vi "ZoneBlue rotatePlace.vi"   [LabVIEW 2019]
uses:
  Global Var.vi
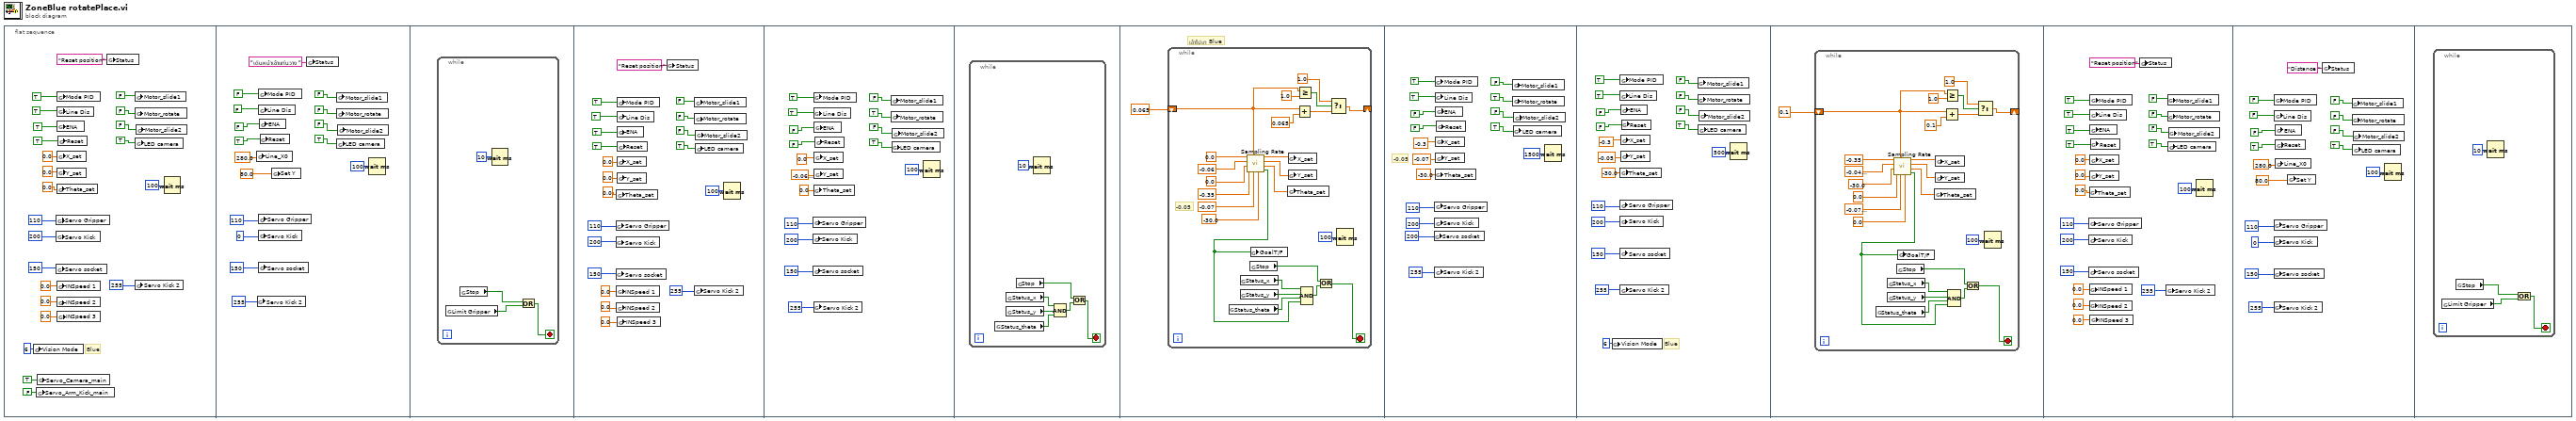
[diagram p0: block diagram]
diagram:
  n1 = flat-sequence {
    frame #0 {
      # "Blue"
      n2 = global write "Global Var.vi" "Vision Mode"(i16 6 ("Vision Mode")) -> ()
      n3 = global write "Global Var.vi" "Servo_Arm_Kick_main"(FALSE ("Mode PID")) -> ()
      n4 = global write "Global Var.vi" "Servo_Camera_main"(TRUE ("Mode PID")) -> ()
      n5 = global write "Global Var.vi" "Servo Gripper"(u8 110 ("Servo Camera")) -> ()
      n6 = global write "Global Var.vi" "Servo Kick"(u8 200 ("Servo Camera")) -> ()
      n7 = global write "Global Var.vi" "Servo socket"(u8 150 ("Servo Camera")) -> ()
      n8 = global write "Global Var.vi" "Theta_set"(0.0 ("Theta_set")) -> ()
      n9 = global write "Global Var.vi" "INSpeed 1"(0.0 ("X_set")) -> ()
      n10 = global write "Global Var.vi" "INSpeed 2"(0.0 ("Y_set")) -> ()
      n11 = global write "Global Var.vi" "Mode PID"(TRUE ("Mode PID")) -> ()
      n12 = global write "Global Var.vi" "Line Dis"(TRUE ("Mode PID")) -> ()
      n13 = global write "Global Var.vi" "ENA"(TRUE ("ENA")) -> ()
      n14 = global write "Global Var.vi" "X_set"(0.0 ("X_set")) -> ()
      n15 = global write "Global Var.vi" "Y_set"(0.0 ("Y_set")) -> ()
      n16 = global write "Global Var.vi" "INSpeed 3"(0.0 ("Theta_set")) -> ()
      n17 = global write "Global Var.vi" "Reset"(TRUE ("ENA")) -> ()
      n18 = global write "Global Var.vi" "Status"("Reset position" ("Status")) -> ()
      n19 = global write "Global Var.vi" "Motor_slide1"(FALSE ("Mode PID")) -> ()
      n20 = global write "Global Var.vi" "Motor_rotate"(FALSE ("ENA")) -> ()
      n21 = global write "Global Var.vi" "Servo Kick 2"(u8 255 ("Servo Camera")) -> ()
      n22 = global write "Global Var.vi" "LED camera"(TRUE ("LED camera")) -> ()
      n23 = global write "Global Var.vi" "Motor_slide2"(FALSE ("ENA")) -> ()
      n24 = Wait (ms)(milliseconds to wait=u32 100) -> ()  [unwired: 1 out]
    }
    frame #1 {
      n25 = global write "Global Var.vi" "Line_X0"(280.0 ("Y_set")) -> ()
      n26 = global write "Global Var.vi" "Servo Kick 2"(u8 255 ("Servo Camera")) -> ()
      n27 = global write "Global Var.vi" "Servo Gripper"(u8 110 ("Servo Camera")) -> ()
      n28 = global write "Global Var.vi" "Servo Kick"(u8 0 ("Servo Camera")) -> ()
      n29 = global write "Global Var.vi" "Servo socket"(u8 150 ("Servo Camera")) -> ()
      n30 = global write "Global Var.vi" "Mode PID"(FALSE ("Mode PID")) -> ()
      n31 = global write "Global Var.vi" "Line Dis"(FALSE ("Mode PID")) -> ()
      n32 = global write "Global Var.vi" "ENA"(FALSE ("ENA")) -> ()
      n33 = global write "Global Var.vi" "Reset"(TRUE ("ENA")) -> ()
      n34 = global write "Global Var.vi" "Set Y"(80.0 ("Y_set")) -> ()
      n35 = global write "Global Var.vi" "Status"("เดินหน้าเข้าแท่นวาง " ("Status")) -> ()
      n36 = global write "Global Var.vi" "Motor_slide1"(FALSE ("Mode PID")) -> ()
      n37 = global write "Global Var.vi" "Motor_rotate"(FALSE ("ENA")) -> ()
      n38 = global write "Global Var.vi" "LED camera"(TRUE ("LED camera")) -> ()
      n39 = global write "Global Var.vi" "Motor_slide2"(FALSE ("ENA")) -> ()
      n40 = Wait (ms)(milliseconds to wait=u32 100) -> ()  [unwired: 1 out]
    }
    frame #2 {
      n41 = while {
        stop <- w42 stop-if-true
        n42 = global read "Global Var.vi" "Limit Gripper"() -> (w40:bool)
        n43 = global read "Global Var.vi" "Stop"() -> (w41:bool)
        n44 = Wait (ms)(milliseconds to wait=u32 10) -> ()  [unwired: 1 out]
        n45 = Or(x=w41, y=w40) -> (x .or. y?=w42:bool)
      }
    }
    frame #3 {
      n46 = global write "Global Var.vi" "Servo Gripper"(u8 110 ("Servo Camera")) -> ()
      n47 = global write "Global Var.vi" "Servo Kick"(u8 200 ("Servo Camera")) -> ()
      n48 = global write "Global Var.vi" "Servo socket"(u8 150 ("Servo Camera")) -> ()
      n49 = global write "Global Var.vi" "Theta_set"(0.0 ("Theta_set")) -> ()
      n50 = global write "Global Var.vi" "INSpeed 1"(0.0 ("X_set")) -> ()
      n51 = global write "Global Var.vi" "INSpeed 2"(0.0 ("Y_set")) -> ()
      n52 = global write "Global Var.vi" "Mode PID"(TRUE ("Mode PID")) -> ()
      n53 = global write "Global Var.vi" "Line Dis"(TRUE ("Mode PID")) -> ()
      n54 = global write "Global Var.vi" "ENA"(TRUE ("ENA")) -> ()
      n55 = global write "Global Var.vi" "X_set"(0.0 ("X_set")) -> ()
      n56 = global write "Global Var.vi" "Y_set"(0.0 ("Y_set")) -> ()
      n57 = global write "Global Var.vi" "INSpeed 3"(0.0 ("Theta_set")) -> ()
      n58 = global write "Global Var.vi" "Reset"(TRUE ("ENA")) -> ()
      n59 = global write "Global Var.vi" "Status"("Reset position" ("Status")) -> ()
      n60 = global write "Global Var.vi" "Motor_slide1"(FALSE ("Mode PID")) -> ()
      n61 = global write "Global Var.vi" "Motor_rotate"(FALSE ("ENA")) -> ()
      n62 = global write "Global Var.vi" "Servo Kick 2"(u8 255 ("Servo Camera")) -> ()
      n63 = global write "Global Var.vi" "LED camera"(TRUE ("LED camera")) -> ()
      n64 = global write "Global Var.vi" "Motor_slide2"(FALSE ("ENA")) -> ()
      n65 = Wait (ms)(milliseconds to wait=u32 100) -> ()  [unwired: 1 out]
    }
    frame #4 {
      n66 = global write "Global Var.vi" "Servo Gripper"(u8 110 ("Servo Camera")) -> ()
      n67 = global write "Global Var.vi" "Servo Kick"(u8 200 ("Servo Camera")) -> ()
      n68 = global write "Global Var.vi" "Servo socket"(u8 150 ("Servo Camera")) -> ()
      n69 = global write "Global Var.vi" "Mode PID"(TRUE ("Mode PID")) -> ()
      n70 = global write "Global Var.vi" "Line Dis"(TRUE ("Mode PID")) -> ()
      n71 = global write "Global Var.vi" "Theta_set"(0.0 ("Theta_set")) -> ()
      n72 = global write "Global Var.vi" "Servo Kick 2"(u8 255 ("Servo Camera")) -> ()
      n73 = global write "Global Var.vi" "ENA"(FALSE ("ENA")) -> ()
      n74 = global write "Global Var.vi" "X_set"(0.0 ("X_set")) -> ()
      n75 = global write "Global Var.vi" "Y_set"(-0.060000000000000005 ("Y_set")) -> ()
      n76 = global write "Global Var.vi" "Reset"(FALSE ("ENA")) -> ()
      n77 = global write "Global Var.vi" "Motor_slide1"(FALSE ("Mode PID")) -> ()
      n78 = global write "Global Var.vi" "Motor_rotate"(TRUE ("ENA")) -> ()
      n79 = global write "Global Var.vi" "LED camera"(TRUE ("LED camera")) -> ()
      n80 = global write "Global Var.vi" "Motor_slide2"(FALSE ("ENA")) -> ()
      n81 = Wait (ms)(milliseconds to wait=u32 100) -> ()  [unwired: 1 out]
    }
    frame #5 {
      n82 = while {
        stop <- w82 stop-if-true
        n83 = global read "Global Var.vi" "Status_theta"() -> (w84:bool)
        n84 = global read "Global Var.vi" "Status_x"() -> (w85:bool)
        n85 = global read "Global Var.vi" "Status_y"() -> (w86:bool)
        n86 = global read "Global Var.vi" "Stop"() -> (w80:bool)
        n87 = Wait (ms)(milliseconds to wait=u32 10) -> ()  [unwired: 1 out]
        n88 = Compound Arithmetic op=AND(w85, w86, w84) -> (w81:bool)
        n89 = Or(x=w80, y=w81) -> (x .or. y?=w82:bool)
      }
    }
    frame #6 {
      # "เข้าไปเท Blue"
      n90 = while {
        shift-right: [w90] -> _
        shift-left: 0.065 -> [w88]
        stop <- w107 stop-if-true
        # "-0.05"
        n91 = global read "Global Var.vi" "Status_theta"() -> (w109:bool)
        n92 = global read "Global Var.vi" "Status_x"() -> (w110:bool)
        n93 = global read "Global Var.vi" "Status_y"() -> (w111:bool)
        n94 = call "Sampling Rate.vi"("input a1"=-30.0, "input y1"=-0.07, "T(0-1)"=w88, "input x1"=-0.35, "input a0"=0.0, "input y0"=-0.06, "input x0"=0.0) -> ("GoalT/F"=w95:bool, "a_output"=w102:dbl, "y_output"=w103:dbl, "x_output"=w104:dbl)  [unwired: 1 in]
        n95 = global read "Global Var.vi" "Stop"() -> (w105:bool)
        n96 = global write "Global Var.vi" "GoalT/F"(w95) -> ()
        n97 = global write "Global Var.vi" "Theta_set"(w102) -> ()
        n98 = global write "Global Var.vi" "X_set"(w104) -> ()
        n99 = global write "Global Var.vi" "Y_set"(w103) -> ()
        n100 = Add(x=w88, y=0.065) -> (x+y=w93:dbl)
        n101 = Greater Or Equal?(x=w88, y=1.0) -> (x >= y?=w92:bool)
        n102 = Compound Arithmetic op=AND(w110, w111, w109, w95) -> (w106:bool)
        n103 = Or(x=w105, y=w106) -> (x .or. y?=w107:bool)
        n104 = Select(t=1.0, s=w92, f=w93) -> (s? t:f=w90:dbl)
        n105 = Wait (ms)(milliseconds to wait=u32 100) -> ()  [unwired: 1 out]
      }
    }
    frame #7 {
      # "-0.05"
      n106 = global write "Global Var.vi" "Servo socket"(u8 200 ("Servo Camera")) -> ()
      n107 = global write "Global Var.vi" "Servo Gripper"(u8 110 ("Servo Camera")) -> ()
      n108 = global write "Global Var.vi" "Servo Kick"(u8 200 ("Servo Camera")) -> ()
      n109 = global write "Global Var.vi" "Servo Kick 2"(u8 255 ("Servo Camera")) -> ()
      n110 = global write "Global Var.vi" "Mode PID"(TRUE ("Mode PID")) -> ()
      n111 = global write "Global Var.vi" "Line Dis"(TRUE ("Mode PID")) -> ()
      n112 = global write "Global Var.vi" "Theta_set"(-30.0 ("Theta_set")) -> ()
      n113 = global write "Global Var.vi" "ENA"(FALSE ("ENA")) -> ()
      n114 = global write "Global Var.vi" "X_set"(-0.3 ("X_set")) -> ()
      n115 = global write "Global Var.vi" "Y_set"(-0.07 ("Y_set")) -> ()
      n116 = global write "Global Var.vi" "Reset"(FALSE ("ENA")) -> ()
      n117 = global write "Global Var.vi" "Motor_slide1"(FALSE ("Mode PID")) -> ()
      n118 = global write "Global Var.vi" "Motor_rotate"(TRUE ("ENA")) -> ()
      n119 = global write "Global Var.vi" "LED camera"(TRUE ("LED camera")) -> ()
      n120 = global write "Global Var.vi" "Motor_slide2"(FALSE ("ENA")) -> ()
      n121 = Wait (ms)(milliseconds to wait=u32 1500) -> ()  [unwired: 1 out]
    }
    frame #8 {
      # "Blue"
      n122 = global write "Global Var.vi" "Vision Mode"(i16 6 ("Vision Mode")) -> ()
      n123 = global write "Global Var.vi" "Servo Gripper"(u8 110 ("Servo Camera")) -> ()
      n124 = global write "Global Var.vi" "Servo Kick"(u8 200 ("Servo Camera")) -> ()
      n125 = global write "Global Var.vi" "Servo socket"(u8 150 ("Servo Camera")) -> ()
      n126 = global write "Global Var.vi" "Mode PID"(TRUE ("Mode PID")) -> ()
      n127 = global write "Global Var.vi" "Line Dis"(TRUE ("Mode PID")) -> ()
      n128 = global write "Global Var.vi" "Theta_set"(-30.0 ("Theta_set")) -> ()
      n129 = global write "Global Var.vi" "Servo Kick 2"(u8 255 ("Servo Camera")) -> ()
      n130 = global write "Global Var.vi" "ENA"(FALSE ("ENA")) -> ()
      n131 = global write "Global Var.vi" "X_set"(-0.3 ("X_set")) -> ()
      n132 = global write "Global Var.vi" "Y_set"(-0.05 ("Y_set")) -> ()
      n133 = global write "Global Var.vi" "Reset"(FALSE ("ENA")) -> ()
      n134 = global write "Global Var.vi" "Motor_slide1"(FALSE ("Mode PID")) -> ()
      n135 = global write "Global Var.vi" "Motor_rotate"(FALSE ("ENA")) -> ()
      n136 = global write "Global Var.vi" "LED camera"(TRUE ("LED camera")) -> ()
      n137 = global write "Global Var.vi" "Motor_slide2"(FALSE ("ENA")) -> ()
      n138 = Wait (ms)(milliseconds to wait=u32 500) -> ()  [unwired: 1 out]
    }
    frame #9 {
      n139 = while {
        shift-right: [w148] -> _
        shift-left: 0.1 -> [w146]
        stop <- w165 stop-if-true
        n140 = global read "Global Var.vi" "Status_theta"() -> (w167:bool)
        n141 = global read "Global Var.vi" "Status_x"() -> (w168:bool)
        n142 = global read "Global Var.vi" "Status_y"() -> (w169:bool)
        n143 = call "Sampling Rate.vi"("input a1"=0.0, "input y1"=-0.07999999999999999, "T(0-1)"=w146, "input x1"=0.0, "input a0"=-30.0, "input y0"=-0.04999999999999999, "input x0"=-0.35) -> ("GoalT/F"=w153:bool, "a_output"=w160:dbl, "y_output"=w161:dbl, "x_output"=w162:dbl)  [unwired: 1 in]
        n144 = global read "Global Var.vi" "Stop"() -> (w163:bool)
        n145 = global write "Global Var.vi" "GoalT/F"(w153) -> ()
        n146 = global write "Global Var.vi" "Theta_set"(w160) -> ()
        n147 = global write "Global Var.vi" "X_set"(w162) -> ()
        n148 = global write "Global Var.vi" "Y_set"(w161) -> ()
        n149 = Add(x=w146, y=0.1) -> (x+y=w151:dbl)
        n150 = Greater Or Equal?(x=w146, y=1.0) -> (x >= y?=w150:bool)
        n151 = Compound Arithmetic op=AND(w168, w169, w167, w153) -> (w164:bool)
        n152 = Or(x=w163, y=w164) -> (x .or. y?=w165:bool)
        n153 = Select(t=1.0, s=w150, f=w151) -> (s? t:f=w148:dbl)
        n154 = Wait (ms)(milliseconds to wait=u32 100) -> ()  [unwired: 1 out]
      }
    }
    frame #10 {
      n155 = global write "Global Var.vi" "Servo Gripper"(u8 110 ("Servo Camera")) -> ()
      n156 = global write "Global Var.vi" "Servo Kick"(u8 200 ("Servo Camera")) -> ()
      n157 = global write "Global Var.vi" "Servo socket"(u8 150 ("Servo Camera")) -> ()
      n158 = global write "Global Var.vi" "Theta_set"(0.0 ("Theta_set")) -> ()
      n159 = global write "Global Var.vi" "INSpeed 1"(0.0 ("X_set")) -> ()
      n160 = global write "Global Var.vi" "INSpeed 2"(0.0 ("Y_set")) -> ()
      n161 = global write "Global Var.vi" "Mode PID"(TRUE ("Mode PID")) -> ()
      n162 = global write "Global Var.vi" "Line Dis"(TRUE ("Mode PID")) -> ()
      n163 = global write "Global Var.vi" "ENA"(TRUE ("ENA")) -> ()
      n164 = global write "Global Var.vi" "X_set"(0.0 ("X_set")) -> ()
      n165 = global write "Global Var.vi" "Y_set"(0.0 ("Y_set")) -> ()
      n166 = global write "Global Var.vi" "INSpeed 3"(0.0 ("Theta_set")) -> ()
      n167 = global write "Global Var.vi" "Reset"(TRUE ("ENA")) -> ()
      n168 = global write "Global Var.vi" "Status"("Reset position" ("Status")) -> ()
      n169 = global write "Global Var.vi" "Servo Kick 2"(u8 255 ("Servo Camera")) -> ()
      n170 = global write "Global Var.vi" "Motor_slide1"(FALSE ("Mode PID")) -> ()
      n171 = global write "Global Var.vi" "Motor_rotate"(FALSE ("ENA")) -> ()
      n172 = global write "Global Var.vi" "LED camera"(TRUE ("LED camera")) -> ()
      n173 = global write "Global Var.vi" "Motor_slide2"(FALSE ("ENA")) -> ()
      n174 = Wait (ms)(milliseconds to wait=u32 100) -> ()  [unwired: 1 out]
    }
    frame #11 {
      n175 = global write "Global Var.vi" "Servo Gripper"(u8 110 ("Servo Camera")) -> ()
      n176 = global write "Global Var.vi" "Servo Kick"(u8 0 ("Servo Camera")) -> ()
      n177 = global write "Global Var.vi" "Servo socket"(u8 150 ("Servo Camera")) -> ()
      n178 = global write "Global Var.vi" "Servo Kick 2"(u8 255 ("Servo Camera")) -> ()
      n179 = global write "Global Var.vi" "Mode PID"(FALSE ("Mode PID")) -> ()
      n180 = global write "Global Var.vi" "Line Dis"(FALSE ("Mode PID")) -> ()
      n181 = global write "Global Var.vi" "ENA"(FALSE ("ENA")) -> ()
      n182 = global write "Global Var.vi" "Line_X0"(280.0 ("Y_set")) -> ()
      n183 = global write "Global Var.vi" "Reset"(TRUE ("ENA")) -> ()
      n184 = global write "Global Var.vi" "Set Y"(80.0 ("Y_set")) -> ()
      n185 = global write "Global Var.vi" "Status"("Distance " ("Status")) -> ()
      n186 = global write "Global Var.vi" "Motor_slide1"(FALSE ("Mode PID")) -> ()
      n187 = global write "Global Var.vi" "Motor_rotate"(FALSE ("ENA")) -> ()
      n188 = global write "Global Var.vi" "LED camera"(TRUE ("LED camera")) -> ()
      n189 = global write "Global Var.vi" "Motor_slide2"(FALSE ("ENA")) -> ()
      n190 = Wait (ms)(milliseconds to wait=u32 100) -> ()  [unwired: 1 out]
    }
    frame #12 {
      n191 = while {
        stop <- w208 stop-if-true
        n192 = global read "Global Var.vi" "Limit Gripper"() -> (w206:bool)
        n193 = global read "Global Var.vi" "Stop"() -> (w207:bool)
        n194 = Wait (ms)(milliseconds to wait=u32 10) -> ()  [unwired: 1 out]
        n195 = Or(x=w207, y=w206) -> (x .or. y?=w208:bool)
      }
    }
  }
